vi "getPathOfTestVi.vi"() -> (3 "pathOfTestVi":path)   [LabVIEW 2018]
doc: "Get the path of test vi: addComplexOne.vi."
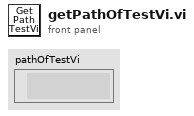
[diagram p1: front panel]
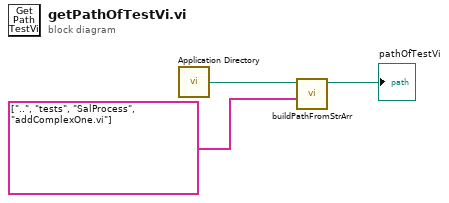
[diagram p0: block diagram]
diagram:
  n1 = call <vilib>:"Application Directory.vi"() -> ("Application Directory"=w2:path)
  n2 = call "buildPathFromStrArr.vi"("String Array"=string[] ["..", "tests", "SalProcess", "addComplexOne.vi"], "Root Path"=w2) -> ("Absolute Path"=→"pathOfTestVi":path)  [unwired: 9 in]
